vi "mlink_led_write.vi"(8 "error in (no error)":errorcluster, 9 "state":bool, 10 "LED":enum8{"None", "D1 (LED1)", "D2 (LED2)"}(ring)=enum."D1 (LED1)", 11 "connection ID":i32=-1) -> (0 "error out":errorcluster, 3 "link_fd out":i32)   [LabVIEW 2009, in "MicroDAQ.lvlib" / "mlink.lvlib"]
doc: "This function sets states of MicroDAQ built in D1 and D2 LEDs."
uses:
  <instrlib>/MicroDAQ/Mlink library wraper/mlink.lvlib
  <instrlib>/MicroDAQ/MLink32.dll
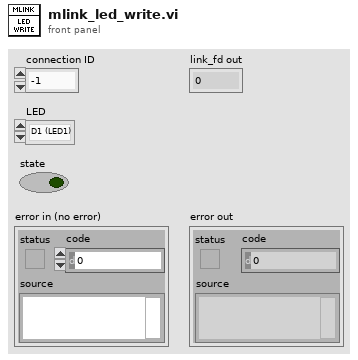
[diagram p1: front panel]
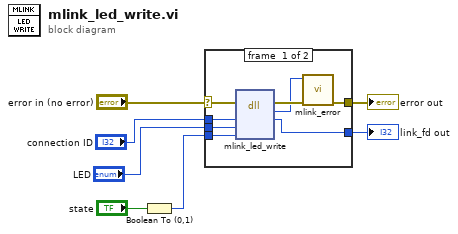
[diagram p0: block diagram]
diagram:
  n1 = Boolean To (0,1)(Boolean="state") -> (0, 1=w2:i16)
  n2 = case shown="No Error" "error in (no error)" {
    selector: "error in (no error)" -> [w13 w17]
    tunnel: "connection ID" -> [w15 w16]
    tunnel: [w14 w16] -> w6
    tunnel: "LED" -> [w12 _]
    tunnel: w2 -> [w11 _]
    tunnel: [w10 w17] -> w1
    frame #0 {
      n3 = dll-call lib="C:/Program Files (x86)/National Instruments/LabVIEW 2009/instr.lib/MicroDAQ/MLink32.dll" fn="mlink_led_write"(error in=w13, "link_fd"=w15, "led"=w12, "state"=w11) -> (error out=w9:errorcluster, "return type"=w8:i32, "link_fd"=w14:i32)  [unwired: 4 in, 1 out]
      n4 = call <instrlib>:"mlink_error.vi"("error in (no error)"=w9, "error code"=w8) -> ("error out"=w10:errorcluster)  [unwired: 9 in]
    }
    frame #1 {
    }
  }
  "link_fd out" <- w6
  "error out" <- w1
